vi "Compose LabVIEW Object - Child - Value.vi"() -> ()   [LabVIEW 2017, in "Composition.Tests.lvlib"]
uses:
  Composition.Tests.lvlib
  Classes/Child/Child.lvclass
  bbe51092-89f6-4f40-b21f-7b28db639aa7.vi
  Composition/Get ClassName From Flattened Object.vi
  <vilib>/Utility/LVClass/Qualified Name Array To Single String.vi
  <vilib>/addons/_JKI Toolkits/Caraya/classes/Assert/Assert.lvclass
  <vilib>/addons/_JKI Toolkits/Caraya/classes/Test/Test.lvclass
panel:
  out "error out":errorcluster
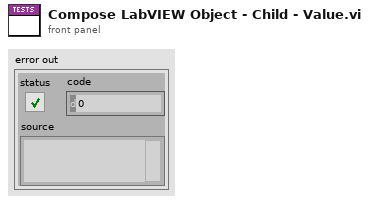
[diagram p1: front panel]
types:
  T1 = cluster{"Major":u16, "Minor":u16, "Fix":u16, "Build":u16}[]
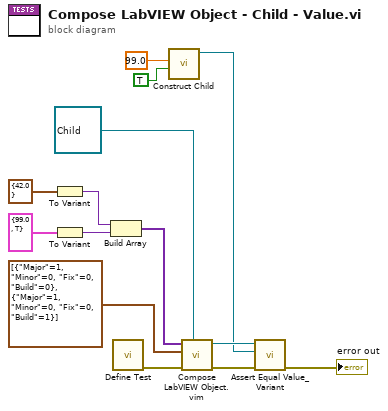
[diagram p0: block diagram]
diagram:
  n1 = To Variant(anything=cluster{dbl} {42.0}) -> (Variant=w10:variant)
  n2 = To Variant(anything=cluster{dbl, bool} {99.0, TRUE}) -> (Variant=w11:variant)
  n3 = Build Array(w10, w11) -> (w8:variant[])
  n4 = call <vilib>:"Define Test.vi"() -> ("error out"=w2:errorcluster)  [unwired: 10 in, 1 out]
  n5 = call "Construct Child.vi"("Ignored"=TRUE, "Offset"=99.0) -> ("Child out"=w3:refnum<class "Child.lvclass">)  [unwired: 8 in, 1 out]
  n6 = call "Compose LabVIEW Object.vim"("Type"=refnum<class "Child.lvclass"> refnum ("Reflection.Tests.lvlib:Child.lvclass"), "error in (no error)"=w2, "Library Versions"=T1 [{"Major"=1, "Minor"=0, "Fix"=0, "Build"=0}, {"Major"=1, "Minor"=0, "Fix"=0, "Build"=1}], "Private Data Clusters"=w8) -> ("error out"=w1:errorcluster, "LabVIEW Object"=w4:refnum<class "Child.lvclass">)  [unwired: 6 in]
  n7 = call <vilib>:"Assert Equal Value_Variant.vi"("error in (no error)"=w1, "Actual"=w3, "Expected"=w4) -> ("error out"=→"error out":errorcluster)  [unwired: 7 in, 1 out]
